vi "Update Table with Measurmeents.vi"(8 "error in (no error)":errorcluster, 9 "Sample":bool, 10 "AI Chan Avg.":string[](array[string]), 11 "MulticolumnListbox in":refnum<vi>) -> (0 "error out":errorcluster, 3 "MulticolumnListbox out":refnum<vi>)   [LabVIEW 2017]
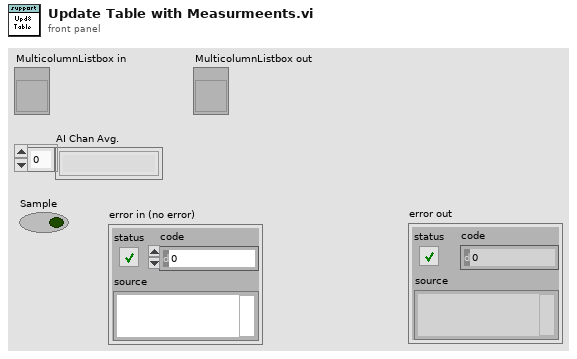
[diagram p1: front panel]
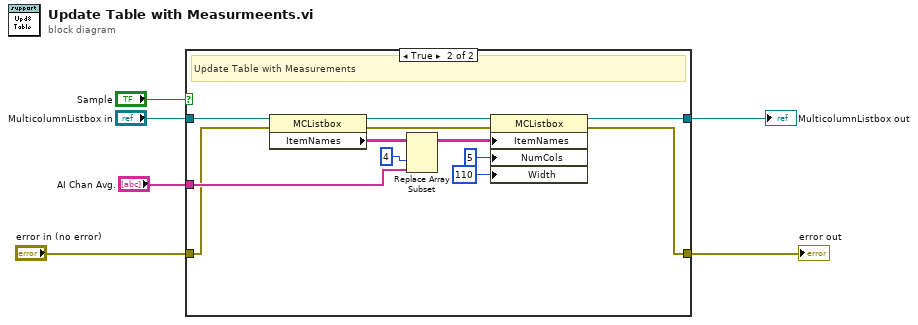
[diagram p0: block diagram]
diagram:
  n1 = case shown="True" "Sample" {
    tunnel: [w8 w20] -> w3
    tunnel: "AI Chan Avg." -> [_ w19]
    tunnel: "MulticolumnListbox in" -> [w8 w17]
    tunnel: [w7 w11] -> w2
    tunnel: "error in (no error)" -> [w7 w13]
    frame False {
    }
    frame True {
      # "Update Table with Measurements"
      n2 = property on="Property Node" class="MCListbox"(reference=w17, error in=w13) -> (reference out=w18:refnum<vi>, error out=w12:errorcluster, "ItemNames"=w14:string[][])
      n3 = Replace Array Subset(array=w14, new element=w19, index (col)=4 ("disabled index (col)")) -> (w15:string[][])  [unwired: 1 in]
      n4 = property on="Property Node" class="MCListbox"(reference=w18, error in=w12, "ItemNames"=w15, "NumCols"=u32 5 ("Number of Columns"), "Width"=u32 110 ("Active Cell:Cell Size:Width")) -> (reference out=w20:refnum<vi>, error out=w11:errorcluster)
    }
  }
  "MulticolumnListbox out" <- w3
  "error out" <- w2
